vi "Shoot.vi"(11 "Balls":u32=10) -> (3 "Shooter time out":u32)   [LabVIEW 2016]
uses:
  Robot Global Data.vi
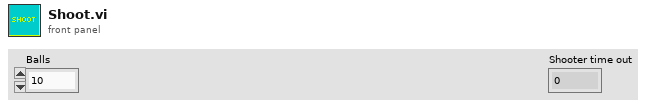
[diagram p1: front panel]
types:
  T1 = typedef "WPI_MotorControlDeviceRef.ctl" = cluster{"DeviceStatus":errorcluster, "Type":T2, "PWM":cluster{"PWM Channel":T3, "DeadBand":T4}, "CAN":cluster{"Device Number":u8, "SetOutput VI Ref":variant, "GetOutput VI Ref":variant, "Enable VI Ref":variant, "Disable VI Ref":variant, "Data":variant}, "Invert":bool}
  T2 = typedef "WPI_MotorControlType.ctl" = enum16{"PWM", "CAN"}
  T3 = typedef "FPGA_DIOPWMChannel.ctl" = enum8{"PWM 0", "PWM 1", "PWM 2", "PWM 3", "PWM 4", "PWM 5", "PWM 6", "PWM 7", "PWM 8", "PWM 9", "PWM MXP 0", "PWM MXP 1", "PWM MXP 2", "PWM MXP 3", "PWM MXP 4", "PWM MXP 5", "PWM MXP 6", "PWM MXP 7", "PWM MXP 8", "PWM MXP 9", "Invalid"}
  T4 = typedef "WPI_PWMDeadband.ctl" = cluster{"Name":string, "maxPositivePwm":i32, "minPositivePwm":i32, "centerPwm":i32, "maxNegativePwm":i32, "minNegativePwm":i32, "angularRange":u16}
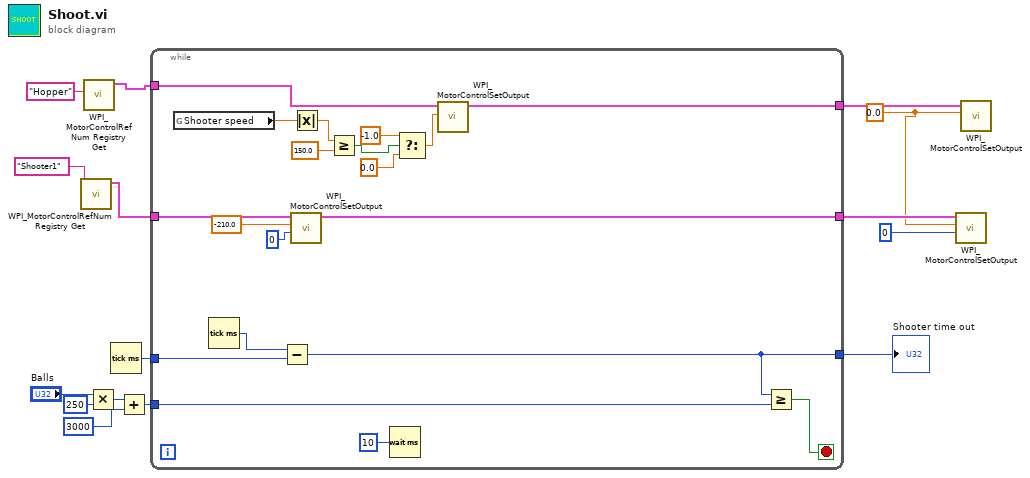
[diagram p0: block diagram]
diagram:
  w12 = 0.0 ("Output")
  n1 = call <vilib>:"WPI_MotorControlRefNum Registry Get.vi"("refnum name"="Shooter1") -> ("MotorControlDevRef"=w7:T1)  [unwired: 9 in, 1 out]
  n2 = call <vilib>:"WPI_MotorControlRefNum Registry Get.vi"("refnum name"="Hopper") -> ("MotorControlDevRef"=w8:T1)  [unwired: 9 in, 1 out]
  n3 = Multiply(x="Balls", y=u32 250) -> (x*y=w3:u32)
  n4 = Tick Count (ms)() -> (millisecond timer value=w15:u32)
  n5 = Add(x=w3, y=u32 3000) -> (x+y=w1:u32)
  n6 = while {
    tunnel: w8 -> [w23]
    tunnel: [w22] -> w14
    tunnel: w7 -> [w21]
    tunnel: [w18] -> w13
    tunnel: w15 -> [w34]
    tunnel: [w17] -> w6
    tunnel: w1 -> [w16]
    stop <- w32 stop-if-true
    n7 = global read "Robot Global Data.vi" "Shooter speed"() -> (w25:dbl)
    n8 = Tick Count (ms)() -> (millisecond timer value=w33:u32)
    n9 = Subtract(x=w33, y=w34) -> (x-y=w17:u32)
    n10 = call <vilib>:"WPI_MotorControlSetOutput.vi"("options"=u8 0, "Output"=-210.0, "MotorControlDevRef"=w21) -> ("MotorControlDevRef"=w18:T1)  [unwired: 6 in, 2 out]
    n11 = Absolute Value(x=w25) -> (abs(x)=w24:dbl)
    n12 = Greater Or Equal?(x=w24, y=150.0) -> (x >= y?=w30:bool)
    n13 = Wait (ms)(milliseconds to wait=u32 10) -> ()  [unwired: 1 out]
    n14 = Select(t=-1.0, s=w30, f=0.0) -> (s? t:f=w27:dbl)
    n15 = call <vilib>:"WPI_MotorControlSetOutput.vi"("Output"=w27, "MotorControlDevRef"=w23) -> ("MotorControlDevRef"=w22:T1)  [unwired: 7 in, 2 out]
    n16 = Greater Or Equal?(x=w17, y=w16) -> (x >= y?=w32:bool)
  }
  "Shooter time out" <- w6
  n17 = call <vilib>:"WPI_MotorControlSetOutput.vi"("options"=u8 0, "Output"=w12, "MotorControlDevRef"=w13) -> ()  [unwired: 6 in, 3 out]
  n18 = call <vilib>:"WPI_MotorControlSetOutput.vi"("Output"=w12, "MotorControlDevRef"=w14) -> ()  [unwired: 7 in, 3 out]
